vi "Open Build.vi"(7 "TargetItem Refnum":refnum<vi>, 8 "error in (no error)":errorcluster, 9 "Build specification name":string, 10 "Build object selector":T1=enum."EXE", 11 "Project Refnum":refnum<vi>) -> (0 "error out":errorcluster, 3 "NI_AB_API_Build out":refnum<class "NI_AB_API_Build.lvclass">)   [LabVIEW 2020, in "NI_AB_API_Build.lvclass"]
uses:
  <vilib>/AppBuilder/AB_API/Build/NI_AB_API_Build.lvclass
  <vilib>/AppBuilder/AB_API/Build/NI_AB_API_Build.lvclass/NI_AB_API_Build.ctl
  <vilib>/AppBuilder/AB_Classes/Build/AB_Build.lvclass
  <vilib>/AppBuilder/AB_API/common/AB_API Build Object Selector.ctl
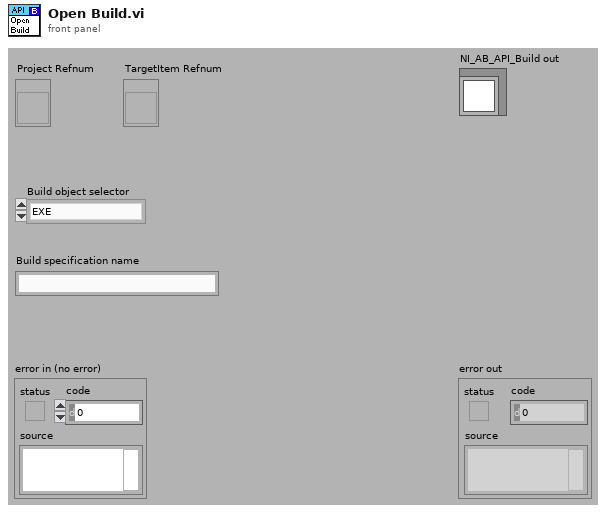
[diagram p1: front panel]
types:
  T1 = typedef "AB_API Build Object Selector.ctl" = enum16{"Source Distribution", "Deployable Source Distribution", "DLL", "EXE", "Packed Library", "Deployable Packed Library", "RT EXE", ".NET Interop Assembly"}
  T2 = typedef "AB_API Build Object Type.ctl" = enum16{"Source Distribution", "DLL", "EXE", "Installer", "Zip File", "RESTful WS", "RTEXE", "Packed Library", "C Generation ", ".NET Interop Assembly"}
  T3 = typedef "ItemRef.ctl" = u64
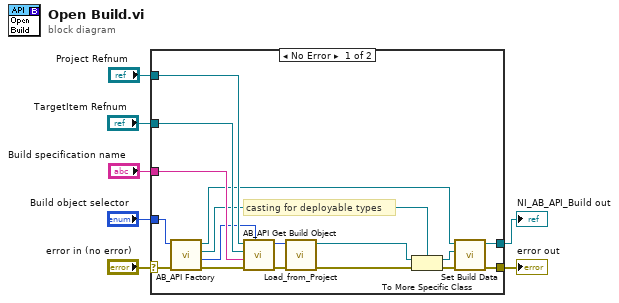
[diagram p0: block diagram]
diagram:
  n1 = case shown="No Error" "error in (no error)" {
    selector: "error in (no error)" -> [w9 w25]
    tunnel: [w18 w25] -> w6
    tunnel: [w19 _] -> w5
    tunnel: "Project Refnum" -> [w22 _]
    tunnel: "TargetItem Refnum" -> [w21 _]
    tunnel: "Build specification name" -> [w20 _]
    tunnel: "Build object selector" -> [w13 _]
    frame No Error {
      # "casting for deployable types"
      n2 = call <vilib>:"AB_API Factory.vi"("error in (no error)"=w9, "Build object selector"=w13) -> ("error out"=w8:errorcluster, "Build object type"=w10:T2, "Build"=w11:refnum<class "AB_Build.lvclass">, "API"=w12:refnum<class "NI_AB_API_Build.lvclass">)  [unwired: 6 in]
      n3 = call <vilib>:"AB_API Get Build Object.vi"("Build object type"=w10, "error in (no error)"=w8, "Build spec name"=w20, "TargetItem Refnum"=w21, "Project Refnum"=w22) -> ("error out"=w23:errorcluster, "Build Object"=w24:T3)  [unwired: 5 in]
      n4 = call <vilib>:"Load_from_Project.vi"("error in (no error)"=w23, "Object"=w24) -> ("error out"=w15:errorcluster, "Build out"=w17:refnum<class "AB_Build.lvclass">)  [unwired: 8 in]
      n5 = To More Specific Class(target class=w11, reference=w17, error in=w15) -> (specific class reference=w16:refnum<class "AB_Build.lvclass">, error out=w14:errorcluster)
      n6 = call <vilib>:"Set Build Data.vi"("error in (no error)"=w14, "AB_Build.lvclass"=w16, "NI_AB_API_Build in"=w12) -> ("error out"=w18:errorcluster, "NI_AB_API_Build out"=w19:refnum<class "NI_AB_API_Build.lvclass">)  [unwired: 7 in]
    }
    frame Error {
    }
  }
  "error out" <- w6
  "NI_AB_API_Build out" <- w5
